vi "YAFTAF_Destructor.vi"(8 "ErrorIn":errorcluster, 10 "CmdData":variant, 11 "LocalIn":refnum<class>) -> (0 "ErrorOut":errorcluster, 2 "ReplyData":variant, 3 "LocalIn":refnum<class>, 4 "Exit":bool)   [LabVIEW 2021, in "YAFTAF.lvclass"]
uses:
  YAFTAF.lvclass
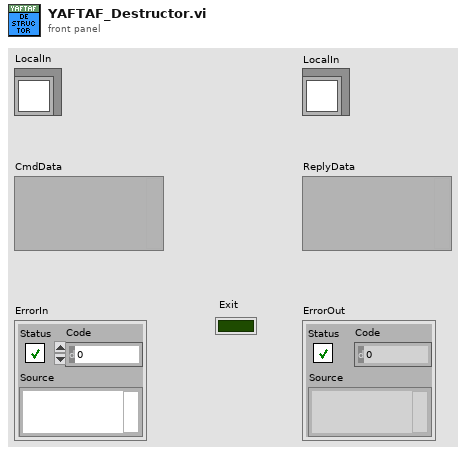
[diagram p1: front panel]
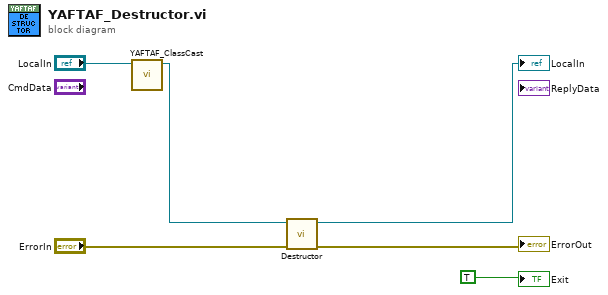
[diagram p0: block diagram]
diagram:
  n1 = call "YAFTAF_ClassCast.vi"("LocalIn"="LocalIn") -> ("LocalOut"=w2:refnum<class "YAFTAF.lvclass">)  [unwired: 10 in]
  n2 = call-dynamic "Destructor.vi"("ErrorIn"="ErrorIn", "ObjectIn"=w2) -> ("ErrorOut"=→"ErrorOut":errorcluster, "ObjectOut"=→"LocalIn":refnum<class "YAFTAF.lvclass">)  [unwired: 8 in]
  "Exit" <- TRUE
